vi "single action cancellable.vi"() -> ()   [LabVIEW 2013]
uses:
  result/result.lvclass
  standard action/wait action/wait action.lvclass
  dispatcher/pool sizes.ctl
  dispatcher/execution system.ctl
  task/task.lvclass/task.ctl
  standard tokens/cancel token/cancel token.lvclass
  result/result.lvclass/result.ctl
  result/get data.vi
  result/get error.vi
  result/get generating action.vi
  result/get owning task.vi
  result/get subresults.vi
  dispatcher/thread pool.lvclass
  standard reporters/event reporter/event reporter.lvclass
  standard tasks/function task/function task.lvclass
  task/task.lvclass
panel:
  out "time to cancel":u32
  out "subresults":refnum<class "result.lvclass">[](array[class])
  out "owning task":string
  out "generating action":string
  out "error":errorcluster
  out "data":variant
  out "Time":u32
  out "result":refnum<class "result.lvclass">
  out "error out":errorcluster
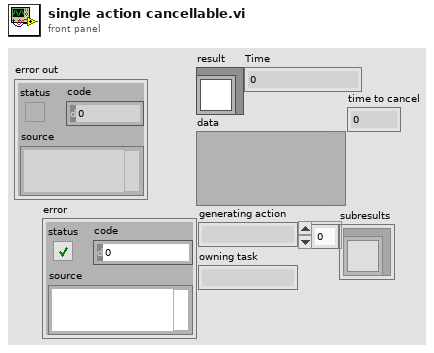
[diagram p1: front panel]
types:
  T1 = typedef "thread pool.lvclass/execution system.ctl" = enum32{"user interface", "standard", "instrument i/o", "data acquisition", "other 1", "other 2"}
  T2 = typedef "thread pool.lvclass/pool sizes.ctl" = cluster{"UI thread":u8, "standard":u8, "instrument I/O":u8, "data acquisition":u8, "other 1":u8, "other 2":u8}
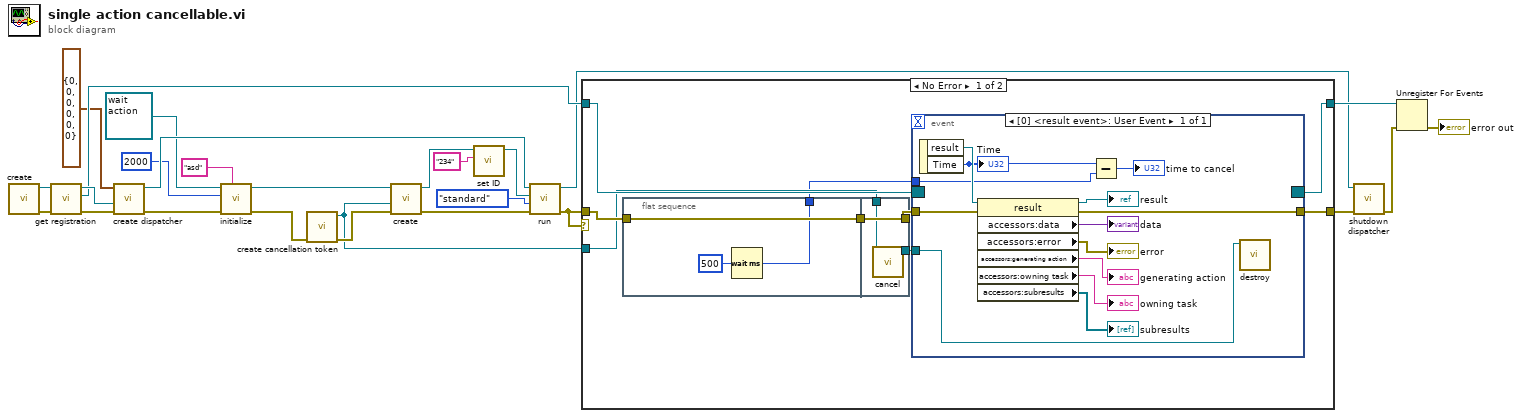
[diagram p0: block diagram]
diagram:
  n1 = call "create.vi"() -> ("error out"=w20:errorcluster, "event reporter out"=w21:refnum<class "event reporter.lvclass">)  [unwired: 10 in]
  n2 = call "get registration.vi"("error in"=w20, "event reporter in"=w21) -> ("error out"=w18:errorcluster, "result registration"=w17:refnum<event-registration>, "event reporter out"=w19:refnum<class "event reporter.lvclass">)  [unwired: 7 in]
  n3 = call "create dispatcher.vi"("error in"=w18, "default reporter"=w19, "initial pool sizes"=T2 {"UI thread"=0, "standard"=0, "instrument I/O"=0, "data acquisition"=0, "other 1"=0, "other 2"=0}) -> ("error out"=w23:errorcluster, "dispatcher"=w25:refnum<data-value>)  [unwired: 7 in]
  n4 = call-dynamic "initialize.vi"("action name"="asd", "error in"=w23, "parameters"=2000, "action in"=refnum<class "wait action.lvclass"> refnum ("wait action.lvclass")) -> ("error out"=w3:errorcluster, "action out"=w11:refnum<class "wait action.lvclass">)  [unwired: 6 in]
  n5 = call "create cancellation token.vi"("error in"=w3) -> ("error out"=w2:errorcluster, "cancel token out"=w1:refnum<class "cancel token.lvclass">)  [unwired: 9 in]
  n6 = call "create.vi"("task token"=w1, "action"=w11) -> ("function task out"=w10:refnum<class "function task.lvclass">)  [unwired: 9 in]
  n7 = call "set ID.vi"("ID"="234", "task in"=w10) -> ("task out"=w9:refnum<class "function task.lvclass">)  [unwired: 9 in]
  n8 = call "run.vi"("error in"=w2, "execution system"=execution_system."standard", "task"=w9, "dispatcher"=w25) -> ("error out"=w6:errorcluster, "dispatcher out"=w15:refnum<data-value>)  [unwired: 6 in]
  n9 = case shown="No Error" w6 {
    tunnel: w17 -> [w34 w55]
    tunnel: [w33 w55] -> w16
    tunnel: [w32 w54] -> w12
    tunnel: w6 -> [w30 w54]
    tunnel: w1 -> [w28 _]
    frame No Error {
      n10 = flat-sequence {
        tunnel: w30 -> [w37]
        tunnel: [w37] -> w29
        tunnel: [w35] -> w26
        tunnel: [w40] -> w31
        tunnel: w29 -> [w40]
        tunnel: w28 -> [w39]
        tunnel: [w38] -> w27
        frame #0 {
          n11 = Wait (ms)(milliseconds to wait=u32 500) -> (millisecond timer value=w35:u32)
        }
        frame #1 {
          n12 = call-dynamic "cancel.vi"("cancel token in"=w39) -> ("cancel token out"=w38:refnum<class "cancel token.lvclass">)  [unwired: 9 in, 1 out]
        }
      }
      n13 = event shown="[0] <result event>: User Event" {
        selector: w34 -> [_]
        dyn-events: [_] -> w33
        timeout: _ -> [_]
        tunnel: [w52] -> w32
        tunnel: w31 -> [w53]
        tunnel: w27 -> [w44]
        tunnel: w26 -> [w42]
        event User Event {
          n14 = event-data() -> ("result"=w51:refnum<class "result.lvclass">, "Time"=w43:u32)  [unwired: 1 in]
          "Time" <- w43
          n15 = property class="result"(reference=w51, error in=w53) -> (reference out=→"result":refnum<class "result.lvclass">, error out=w52:errorcluster, "accessors:data"=→"data":variant, "accessors:error"=→"error":errorcluster, "accessors:generating action"=→"generating action":string, "accessors:owning task"=→"owning task":string, "accessors:subresults"=→"subresults":refnum<class "result.lvclass">[])
          n16 = Subtract(x=w43, y=w42) -> (x-y=→"time to cancel":u32)
          n17 = call-dynamic "destroy.vi"("task token in"=w44) -> ()  [unwired: 10 in, 1 out]
        }
      }
    }
    frame Error {
    }
  }
  n18 = call "shutdown dispatcher.vi"("error in"=w12, "dispatcher"=w15) -> ("error out"=w14:errorcluster)  [unwired: 9 in]
  n19 = Unregister For Events(event registration refnum=w16, error in=w14) -> (error out=→"error out":errorcluster)
